vi "Data_Three Balls.vi"(6 "seed":i32=-1, 10 "noise amplitude":dbl=0.5, 11 "# of points":i32=4000) -> (1 "Classes":i32[](array[numeric]), 3 "Data":dbl[][](array[numeric]))   [LabVIEW 2020]
uses:
  <vilib>/Analysis/NI_AALBase.lvlib
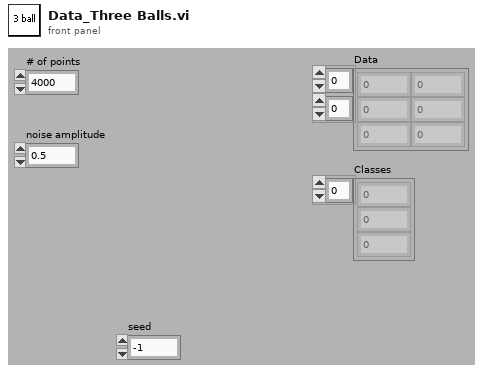
[diagram p1: front panel]
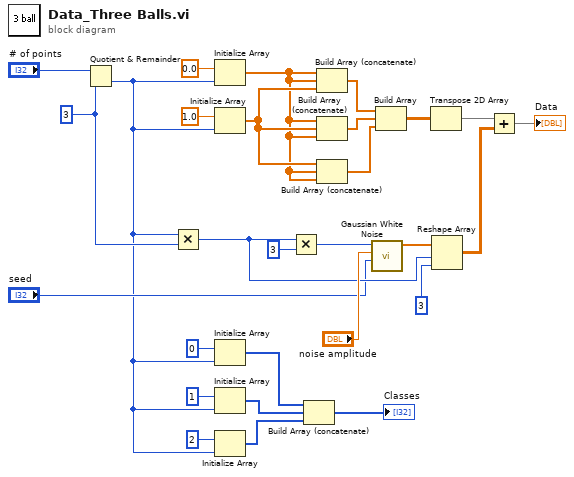
[diagram p0: block diagram]
diagram:
  w17 = 3 ("y")
  n1 = Quotient & Remainder(x="# of points", y=w17) -> (floor(x/y)=w8:i32)  [unwired: 1 out]
  n2 = Multiply(x=w8, y=w17) -> (x*y=w14:i32)
  n3 = Initialize Array(0.0 ("element"), w8) -> (w1:dbl[])
  n4 = Initialize Array(1.0 ("element"), w8) -> (w2:dbl[])
  n5 = Initialize Array(0 ("element"), w8) -> (w7:i32[])
  n6 = Initialize Array(1 ("element"), w8) -> (w6:i32[])
  n7 = Initialize Array(2 ("element"), w8) -> (w5:i32[])
  n8 = Multiply(x=w14, y=3) -> (x*y=w16:i32)
  n9 = Build Array (concatenate)(w7, w6, w5) -> (→"Classes":i32[])
  n10 = Build Array (concatenate)(w1, w1, w2) -> (w23:dbl[])
  n11 = Build Array (concatenate)(w1, w2, w1) -> (w24:dbl[])
  n12 = Build Array (concatenate)(w2, w1, w1) -> (w3:dbl[])
  n13 = call <vilib>:"Gaussian White Noise.vi"("seed"="seed", "standard deviation"="noise amplitude", "samples"=w16) -> ("Gaussian noise pattern"=w28:dbl[])  [unwired: 7 in, 1 out]
  n14 = Build Array(w23, w24, w3) -> (w22:dbl[][])
  n15 = Transpose 2D Array(2D array=w22) -> (transposed array=w20:dbl[][])
  n16 = Reshape Array(w28, w14, 3 ("y")) -> (w21:dbl[][])
  n17 = Add(x=w20, y=w21) -> (x+y=→"Data":dbl[][])
